vi "controlFrequency.vi"(7 "Set":bool, 8 "error in":errorcluster, 9 "Frequency [Hz] in":dbl, 10 "axis in":u8, 11 "connection ID":refnum<k5>) -> (0 "error out":errorcluster, 1 "Frequency [Hz] out":dbl, 2 "axis out":u8, 3 "connection ID":refnum<k5>)   [LabVIEW 2016]
panel:
  in  "Set Command":string="com.attocube.amc.control.setControlFrequency"
  in  "Get Command":string="com.attocube.amc.control.getControlFrequency"
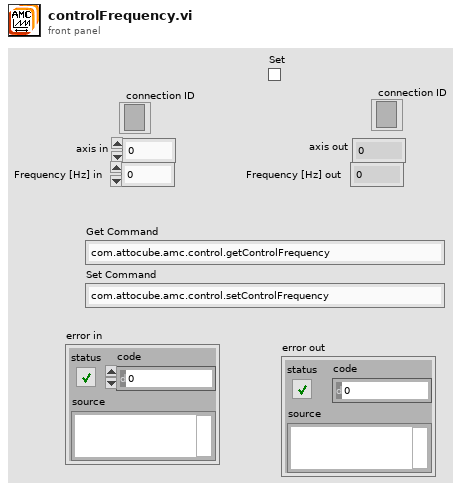
[diagram p1: front panel]
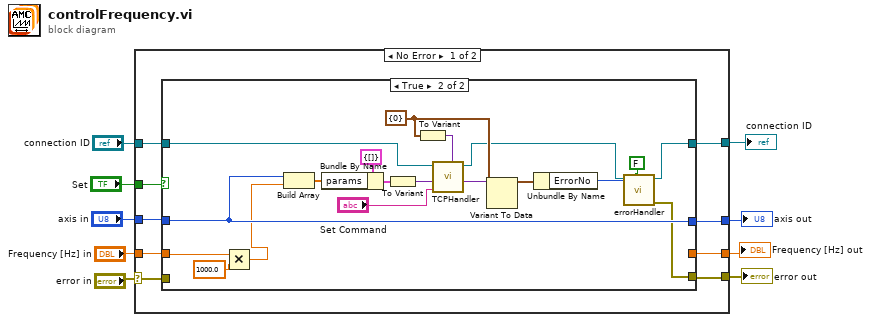
[diagram p0: block diagram]
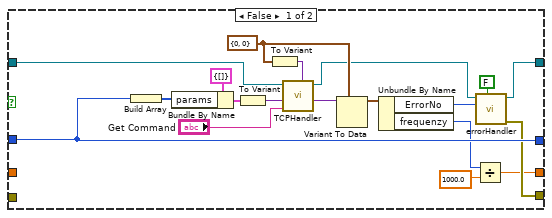
[diagram p2: hidden frame]
diagram:
  n1 = case shown="No Error" "error in" {
    selector: "error in" -> [w14 w60]
    tunnel: "axis in" -> [w16 w58]
    tunnel: [w10 w60] -> w8
    tunnel: [w12 w58] -> w7
    tunnel: "Frequency [Hz] in" -> [w15 w59]
    tunnel: [w11 w59] -> w5
    tunnel: "Set" -> [w17 _]
    tunnel: [w13 w57] -> w3
    tunnel: "connection ID" -> [w18 w57]
    frame No Error {
      n2 = case shown="True" w17 {
        tunnel: [w19 w38] -> w13
        tunnel: w18 -> [w27 w51]
        tunnel: w16 -> [w29 w49]
        tunnel: [w29 w49] -> w12
        tunnel: [w28 w46] -> w10
        tunnel: [w21 _] -> w11
        tunnel: w15 -> [_ w40]
        tunnel: w14 -> [_ _]
        frame False {
          w25 = cluster{"ErrorNo":i16, "frequenzy":i64} {"ErrorNo"=0, "frequenzy"=0} ("input cluster")
          n3 = Build Array(w29) -> (w33:u8[])
          n4 = Bundle By Name(cluster=cluster{"params":i16[]} {"params"=[]} ("input cluster"), "params"=w33) -> (w34:cluster{"params":i16[]})
          n5 = To Variant(anything=w34) -> (Variant=w35:variant)
          n6 = To Variant(anything=w25) -> (Variant=w26:variant)
          n7 = call "TCPHandler.vi"("result Types"=w26, "method"="Get Command", "params"=w35, "connection ID"=w27) -> ("result"=w31:variant, "connection ID"=w20:refnum<k5>)  [unwired: 5 in, 1 out]
          n8 = Variant To Data(type=w25, Variant=w31) -> (data=w36:cluster{"ErrorNo":i16, "frequenzy":i64})  [unwired: 1 in, 1 out]
          n9 = Unbundle By Name(w36) -> ("ErrorNo"=w37:i16, "frequenzy"=w22:i64)
          n10 = Divide(x=w22, y=1000.0) -> (x/y=w21:dbl)
          n11 = call "errorHandler.vi"("show popup"=FALSE, "error number"=w37, "connection ID"=w20) -> ("error out"=w28:errorcluster, "connection ID"=w19:refnum<k5>)  [unwired: 7 in]
        }
        frame True {
          w44 = cluster{"ErrorNo":i16} {"ErrorNo"=0} ("input cluster")
          n12 = Multiply(x=w40, y=1000.0) -> (x*y=w41:dbl)
          n13 = Build Array(w49, w41) -> (w53:dbl[])
          n14 = Bundle By Name(cluster=cluster{"params":i64[]} {"params"=[]} ("input cluster"), "params"=w53) -> (w52:cluster{"params":i64[]})
          n15 = To Variant(anything=w52) -> (Variant=w50:variant)
          n16 = To Variant(anything=w44) -> (Variant=w45:variant)
          n17 = call "TCPHandler.vi"("result Types"=w45, "method"="Set Command", "params"=w50, "connection ID"=w51) -> ("result"=w55:variant, "connection ID"=w39:refnum<k5>)  [unwired: 5 in, 1 out]
          n18 = Variant To Data(type=w44, Variant=w55) -> (data=w48:cluster{"ErrorNo":i16})  [unwired: 1 in, 1 out]
          n19 = Unbundle By Name(w48) -> ("ErrorNo"=w47:i16)
          n20 = call "errorHandler.vi"("show popup"=FALSE, "error number"=w47, "connection ID"=w39) -> ("error out"=w46:errorcluster, "connection ID"=w38:refnum<k5>)  [unwired: 7 in]
        }
      }
    }
    frame Error {
    }
  }
  "error out" <- w8
  "axis out" <- w7
  "Frequency [Hz] out" <- w5
  "connection ID" <- w3
